vi "Teleop Tester.vi"() -> ()   [LabVIEW 2020]
uses:
  <vilib>/Analysis/NI_AALPro.lvlib
  <vilib>/Analysis/coordinate.llb/2D Cartesian Coordinate Rotation (Scalar).vi
panel:
  out "Pose":cluster{dbl, dbl, dbl}
  out "?":picture
  out "RR":bool=TRUE
  # "Teleop Tester:\n\n1.) Plug In Joystick\n2.) Swap out Teleop Emulator VI in\nthe block diagram\n3.) Drive!\n3.) If you lose the robot, click on the\npicture and the robot will move there"
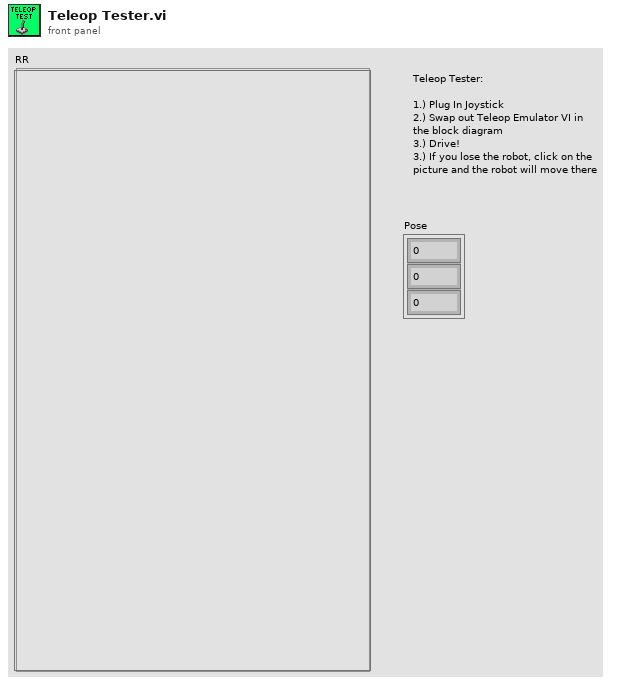
[diagram p1: front panel]
types:
  T1 = typedef "LVPositionTypeDef.ctl" = cluster{"Left":i32, "Top":i32}
  T2 = typedef "LVBoundsTypeDef.ctl" = cluster{"Width":u32, "Height":u32}
  T3 = typedef "Robot Velocities.ctl" = cluster{"X Velocity":dbl, "Y Velocity":dbl, "Rotational \nVelocity":dbl}
  T4 = cluster{"x out":dbl, "y out":dbl, "Rotational \nVelocity":dbl}
  T5 = typedef "LVPoint32TypeDef.ctl" = cluster{"Horizontal":i32, "Vertical":i32}
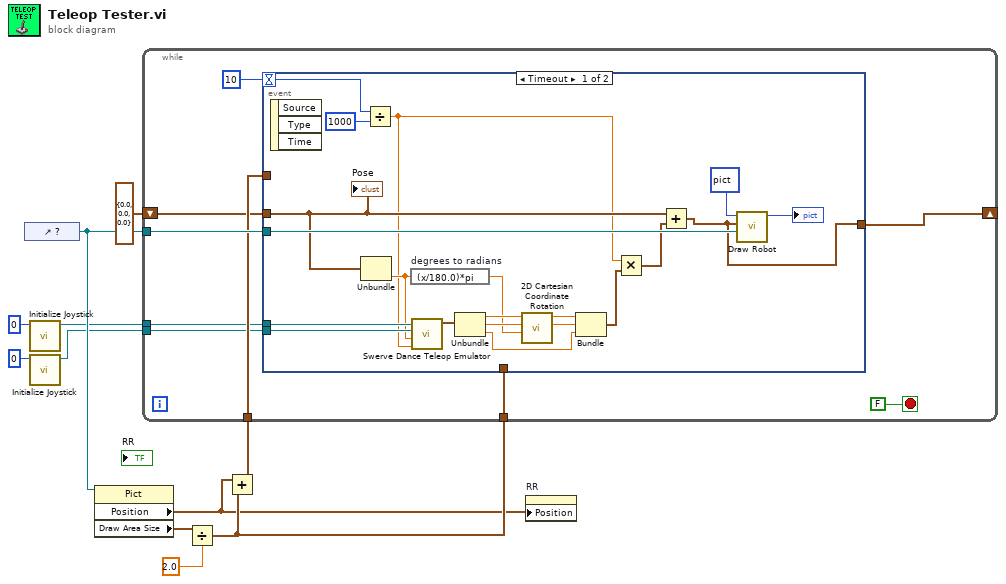
[diagram p0: block diagram]
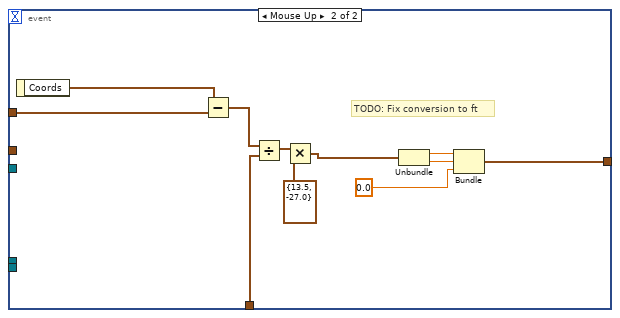
[diagram p2: hidden frame]
diagram:
  n1 = control-ref of="?"() -> (w11:refnum<vi>)
  n2 = call <vilib>:"Initialize Joystick.vi"("device index"=0) -> ("device ID"=w4:refnum<k1>)  [unwired: 9 in, 1 out]
  n3 = call <vilib>:"Initialize Joystick.vi"("device index"=0) -> ("device ID"=w1:refnum<k1>)  [unwired: 9 in, 1 out]
  n4 = property class="Pict"(reference=w11) -> ("Position"=w6:T1, "Draw Area Size"=w10:T2)  [unwired: 1 in, 2 out]
  n5 = Divide(x=w10, y=2.0) -> (x/y=w7:cluster{"Width":dbl, "Height":dbl})
  n6 = Add(x=w6, y=w7) -> (x+y=w8:cluster{dbl, dbl})
  n7 = while {
    tunnel: w11 -> [w18]
    tunnel: w8 -> [w17]
    tunnel: w7 -> [w16]
    shift-right: [w15] -> _
    shift-left: cluster{dbl, dbl, dbl} {0.0, 0.0, 0.0} -> [w14]
    tunnel: w4 -> [w13]
    tunnel: w1 -> [w12]
    stop <- FALSE stop-if-true
    n8 = event shown="[0] Timeout" {
      selector: _ -> [_ _]
      dyn-events: _ -> [_ _]
      timeout: 10 -> [w35 _]
      tunnel: w18 -> [w38 _]
      tunnel: w17 -> [_ w51]
      tunnel: w16 -> [_ w45]
      tunnel: [w37 w41] -> w15
      tunnel: w14 -> [w26 _]
      tunnel: w13 -> [w25 _]
      tunnel: w12 -> [w24 _]
      event Timeout {
        n9 = event-data() -> ()  [unwired: 1 in, 3 out]
        n10 = Unbundle(w26) -> (w22:dbl)  [unwired: 2 out]
        n11 = Divide(x=w35, y=1000) -> (x/y=w21:dbl)
        n12 = expression code="(x/180.0)*pi" "degrees to radians"(w22) -> (w27:dbl)
        n13 = call "Swerve Dance Teleop Emulator.vi"("dt"=w21, "Current Heading"=w22, "Operator ID"=w24, "Driver ID"=w25) -> ("Robot Velocities"=w23:T3)  [unwired: 7 in]
        n14 = Unbundle(w23) -> ("X Velocity"=w33:dbl, "Y Velocity"=w32:dbl, "Rotational \nVelocity"=w29:dbl)
        n15 = call-poly <vilib>:"2D Cartesian Coordinate Rotation.vi"("theta"=w27, "y"=w32, "x"=w33) -> ("y out"=w30:dbl, "x out"=w31:dbl)  [unwired: 6 in, 1 out]
        n16 = Bundle("x out"=w31, "y out"=w30, "Rotational \nVelocity"=w29) -> (w28:T4)  [unwired: 1 in]
        n17 = Multiply(x=w21, y=w28) -> (x*y=w36:T4)
        n18 = Add(x=w26, y=w36) -> (x+y=w37:cluster{dbl, dbl, dbl})
        n19 = call "Draw Robot.vi"("Picture  Reference"=w38, "Pose"=w37, "Picture In"=picture data[5B]) -> ("Picture Out"=→"?":picture)  [unwired: 8 in]
        "Pose" <- w26
      }
      event Mouse Up {
        # "TODO: Fix conversion to ft"
        n20 = event-data() -> ("Coords"=w50:T5)  [unwired: 1 in]
        n21 = Subtract(x=w50, y=w51) -> (x-y=w46:cluster{dbl, dbl})
        n22 = Divide(x=w46, y=w45) -> (x/y=w44:cluster{dbl, dbl})
        n23 = Multiply(x=w44, y=cluster{dbl, dbl} {13.5, -27.0}) -> (x*y=w42:cluster{dbl, dbl})
        n24 = Unbundle(w42) -> (w49:dbl, w48:dbl)
        n25 = Bundle(w49, w48, 0.0) -> (w41:cluster{dbl, dbl, dbl})  [unwired: 1 in]
      }
    }
  }
  n26 = property on="RR" class="Bool (strict)"("Position"=w6) -> ()  [unwired: 2 in, 2 out]
